vi "LSX Set Joystick Dir.vi"(6 "lAD":i32, 7 "lZD":i32, 8 "error in (no error)":errorcluster, 9 "lYD":i32, 10 "lXD":i32, 11 "lLSID":i32) -> (0 "error out":errorcluster, 3 "function return":i32)   [LabVIEW 2018, in "Tango.lvlib"]
doc: "TANGOAPI int TANGOCALL LSX_SetJoystickDir (int lLSID, int lXD, int lYD, int lZD, int lAD);"
uses:
  Tango.lvlib
  SubVIs/Tango_DLL.dll
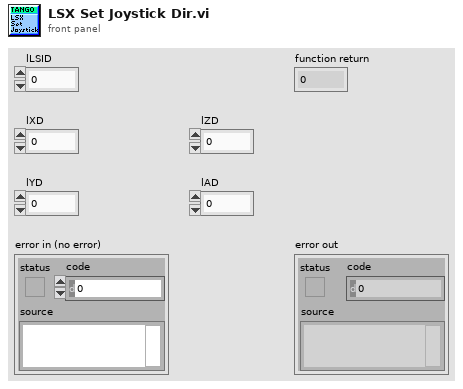
[diagram p1: front panel]
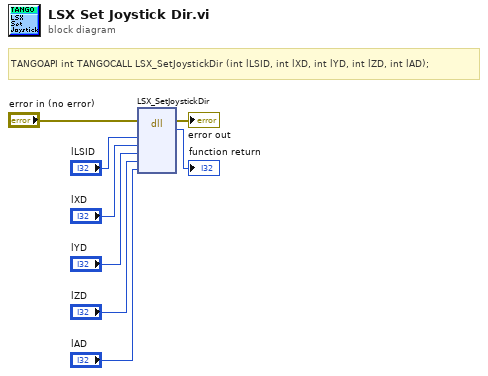
[diagram p0: block diagram]
diagram:
  # "TANGOAPI int TANGOCALL LSX_SetJoystickDir (int lLSID, int lXD, int lYD, int lZD, int lAD);"
  n1 = dll-call lib="C:/Users/Familie/Documents/LabviewIX81/lib/TANGO Stage/SubVIs/Tango_DLL.*" fn="LSX_SetJoystickDir"(error in="error in (no error)", "lLSID"="lLSID", "lXD"="lXD", "lYD"="lYD", "lZD"="lZD", "lAD"="lAD") -> (error out=→"error out":errorcluster, →"function return":i32)  [unwired: 7 in, 1 out]
